vi "Patrick Excess-64.vi"() -> ()   [LabVIEW 2019]
panel:
  out "Boolean array 2":bool[][](array[boolean])=[[FALSE, TRUE, FALSE, FALSE, FALSE, FALSE, FALSE, TRUE, FALSE, FALSE, FALSE, TRUE, FALSE, FALSE, FALSE, FALSE, FALSE, FALSE, FALSE, FALSE, FALSE, FALSE, FALSE, FALSE, FALSE, FALSE, FALSE, FALSE, FALSE, FALSE, FALSE, FALSE], [FALSE, TRUE, FALSE, FALSE, FALSE, FALSE, FALSE, TRUE, FALSE, FALSE, TRUE, FALSE, FALSE, FALSE, FALSE, FALSE, FALSE, FALSE, FALSE, FALSE, FALSE, FALSE, FALSE, FALSE, FALSE, FALSE, FALSE, FALSE, FALSE, FALSE, FALSE, FALSE], [FALSE, TRUE, FALSE, FALSE, FALSE, FALSE, FALSE, TRUE, FALSE, FALSE, TRUE, TRUE, FALSE, FALSE, FALSE, FALSE, FALSE, FALSE, FALSE, FALSE, FALSE, FALSE, FALSE, FALSE, FALSE, FALSE, FALSE, FALSE, FALSE, FALSE, FALSE, FALSE], [TRUE, TRUE, FALSE, FALSE, FALSE, FALSE, FALSE, TRUE, FALSE, FALSE, FALSE, TRUE, FALSE, FALSE, FALSE, FALSE, FALSE, FALSE, FALSE, FALSE, FALSE, FALSE, FALSE, FALSE, FALSE, FALSE, FALSE, FALSE, FALSE, FALSE, FALSE, FALSE], [TRUE, TRUE, FALSE, FALSE, FALSE, FALSE, FALSE, TRUE, FALSE, FALSE, TRUE, FALSE, FALSE, FALSE, FALSE, FALSE, FALSE, FALSE, FALSE, FALSE, FALSE, FALSE, FALSE, FALSE, FALSE, FALSE, FALSE, FALSE, FALSE, FALSE, FALSE, FALSE], [TRUE, TRUE, FALSE, FALSE, FALSE, FALSE, FALSE, TRUE, FALSE, FALSE, TRUE, TRUE, FALSE, FALSE, FALSE, FALSE, FALSE, FALSE, FALSE, FALSE, FALSE, FALSE, FALSE, FALSE, FALSE, FALSE, FALSE, FALSE, FALSE, FALSE, FALSE, FALSE], [FALSE, TRUE, TRUE, FALSE, FALSE, FALSE, FALSE, FALSE, FALSE, TRUE, FALSE, FALSE, FALSE, FALSE, FALSE, FALSE, FALSE, FALSE, FALSE, FALSE, FALSE, FALSE, FALSE, FALSE, FALSE, FALSE, FALSE, FALSE, FALSE, FALSE, FALSE, TRUE], [FALSE, FALSE, TRUE, FALSE, FALSE, FALSE, FALSE, FALSE, FALSE, TRUE, FALSE, FALSE, TRUE, TRUE, FALSE, FALSE, TRUE, TRUE, FALSE, FALSE, TRUE, TRUE, FALSE, FALSE, TRUE, TRUE, FALSE, FALSE, TRUE, TRUE, FALSE, FALSE], [FALSE, FALSE, TRUE, FALSE, FALSE, FALSE, FALSE, FALSE, FALSE, TRUE, FALSE, TRUE, TRUE, FALSE, FALSE, TRUE, TRUE, FALSE, FALSE, TRUE, TRUE, FALSE, FALSE, TRUE, TRUE, FALSE, FALSE, TRUE, TRUE, FALSE, FALSE, TRUE], [FALSE, TRUE, FALSE, FALSE, FALSE, FALSE, FALSE, TRUE, FALSE, FALSE, FALSE, TRUE, TRUE, FALSE, TRUE, TRUE, FALSE, FALSE, TRUE, TRUE, FALSE, FALSE, TRUE, TRUE, FALSE, FALSE, TRUE, TRUE, FALSE, FALSE, TRUE, TRUE], [FALSE, FALSE, FALSE, FALSE, FALSE, FALSE, FALSE, FALSE, FALSE, FALSE, FALSE, FALSE, FALSE, FALSE, FALSE, FALSE, FALSE, FALSE, FALSE, FALSE, FALSE, FALSE, FALSE, FALSE, FALSE, FALSE, FALSE, FALSE, FALSE, FALSE, FALSE, FALSE], [FALSE, TRUE, FALSE, FALSE, FALSE, FALSE, FALSE, TRUE, FALSE, FALSE, FALSE, TRUE, FALSE, FALSE, FALSE, FALSE, FALSE, FALSE, FALSE, FALSE, FALSE, FALSE, FALSE, FALSE, FALSE, FALSE, FALSE, FALSE, FALSE, FALSE, FALSE, FALSE], [FALSE, TRUE, FALSE, FALSE, FALSE, FALSE, FALSE, TRUE, TRUE, FALSE, TRUE, FALSE, FALSE, FALSE, FALSE, FALSE, FALSE, FALSE, FALSE, FALSE, FALSE, FALSE, FALSE, FALSE, FALSE, FALSE, FALSE, FALSE, FALSE, FALSE, FALSE, FALSE], [FALSE, TRUE, FALSE, FALSE, FALSE, FALSE, TRUE, FALSE, FALSE, TRUE, TRUE, FALSE, FALSE, TRUE, FALSE, FALSE, FALSE, FALSE, FALSE, FALSE, FALSE, FALSE, FALSE, FALSE, FALSE, FALSE, FALSE, FALSE, FALSE, FALSE, FALSE, FALSE], [FALSE, TRUE, FALSE, FALSE, FALSE, FALSE, TRUE, TRUE, FALSE, FALSE, TRUE, TRUE, TRUE, TRUE, TRUE, FALSE, FALSE, FALSE, FALSE, FALSE, FALSE, FALSE, FALSE, TRUE, FALSE, FALSE, FALSE, FALSE, FALSE, FALSE, FALSE, FALSE], [FALSE, TRUE, FALSE, FALSE, FALSE, TRUE, FALSE, FALSE, FALSE, FALSE, TRUE, FALSE, FALSE, TRUE, TRUE, TRUE, FALSE, FALSE, FALSE, TRUE, FALSE, FALSE, FALSE, FALSE, FALSE, FALSE, FALSE, FALSE, FALSE, FALSE, FALSE, FALSE], [FALSE, TRUE, FALSE, FALSE, FALSE, TRUE, FALSE, TRUE, FALSE, FALSE, FALSE, TRUE, TRUE, FALSE, FALSE, FALSE, FALSE, TRUE, TRUE, FALSE, TRUE, FALSE, TRUE, FALSE, FALSE, FALSE, FALSE, FALSE, FALSE, FALSE, FALSE, FALSE]]
  out "?":u32=5642402 format="%064b"
  out "Boolean array":bool[](array[boolean])=[FALSE, TRUE, FALSE, FALSE, FALSE, TRUE, FALSE, TRUE, FALSE, FALSE, FALSE, TRUE, TRUE, FALSE, FALSE, FALSE, FALSE, TRUE, TRUE, FALSE, TRUE, FALSE, TRUE, FALSE, FALSE, FALSE, FALSE, FALSE, FALSE, FALSE, FALSE, FALSE]
  in  "Test numbers":u32[](array[numeric])=[1091567616, 1092616192, 1093664768, 3239051264, 3240099840, 3241148416, 1614807041, 541904076, 542742937, 1092301619, 0, 1091567616, 1101004800, 1113849856, 1128136960, 1143410688, 1159227904] format="%032b"
  out "Array":bool[][](array[boolean])=[[FALSE, FALSE, TRUE, TRUE, TRUE, TRUE, TRUE, FALSE], [FALSE, TRUE, FALSE, FALSE, FALSE, FALSE, FALSE, TRUE], [TRUE, FALSE, FALSE, FALSE, TRUE, FALSE, FALSE, TRUE], [FALSE, FALSE, TRUE, TRUE, FALSE, TRUE, TRUE, TRUE], [FALSE, TRUE, FALSE, FALSE, TRUE, FALSE, TRUE, TRUE], [TRUE, TRUE, FALSE, FALSE, FALSE, TRUE, TRUE, FALSE], [TRUE, FALSE, TRUE, FALSE, FALSE, TRUE, TRUE, TRUE], [TRUE, TRUE, TRUE, TRUE, FALSE, TRUE, FALSE, FALSE]]
  out "8 bytes":u8[](array[numeric])=[62, 65, 137, 55, 75, 198, 167, 244] format="%08b"
  out "result":dbl[](array[numeric])=[1.0, 2.0, 3.0, -1.0, -2.0, -3.0, 8.507061201264422e+37, inf, inf, 1.6999998092651367, nan, 1.0, 10.0, 100.0, 992.0625, 10000.0, 100000.0]
  # "https://boolean.klaasholwerda.nl/interface/bnf/gdsformat.html#datatypes"
  # "01000001000100000000000000000000 = 1\n01000001001000000000000000000000 = 2\n01000001001100000000000000000000 = 3\n11000001000100000000000000000000 = -1\n11000001001000000000000000000000 = -2\n11000001001100000000000000000000 = -3\n0100000010000000000000000000000 = 0 .5\n0100000010011001100110011001100 = 1 .6\n0100000010110011001100110011001 = 1 .7\n01000001000110000000000000000000 = 1.5\n01000001000110011001100110011001 = 1.6\n01000001000110110011001100110011 = 1.7\n00000000000000000000000000000000 = 0\n01000001000100000000000000000000 = 1\n01000001101000000000000000000000 = 10\n01000010011001000000000000000000 = 100\n01000011001111100000000100000000 = 1000\n01000100001001110001000000000000 = 10000\n01000101000110000110101000000000 = 100000"
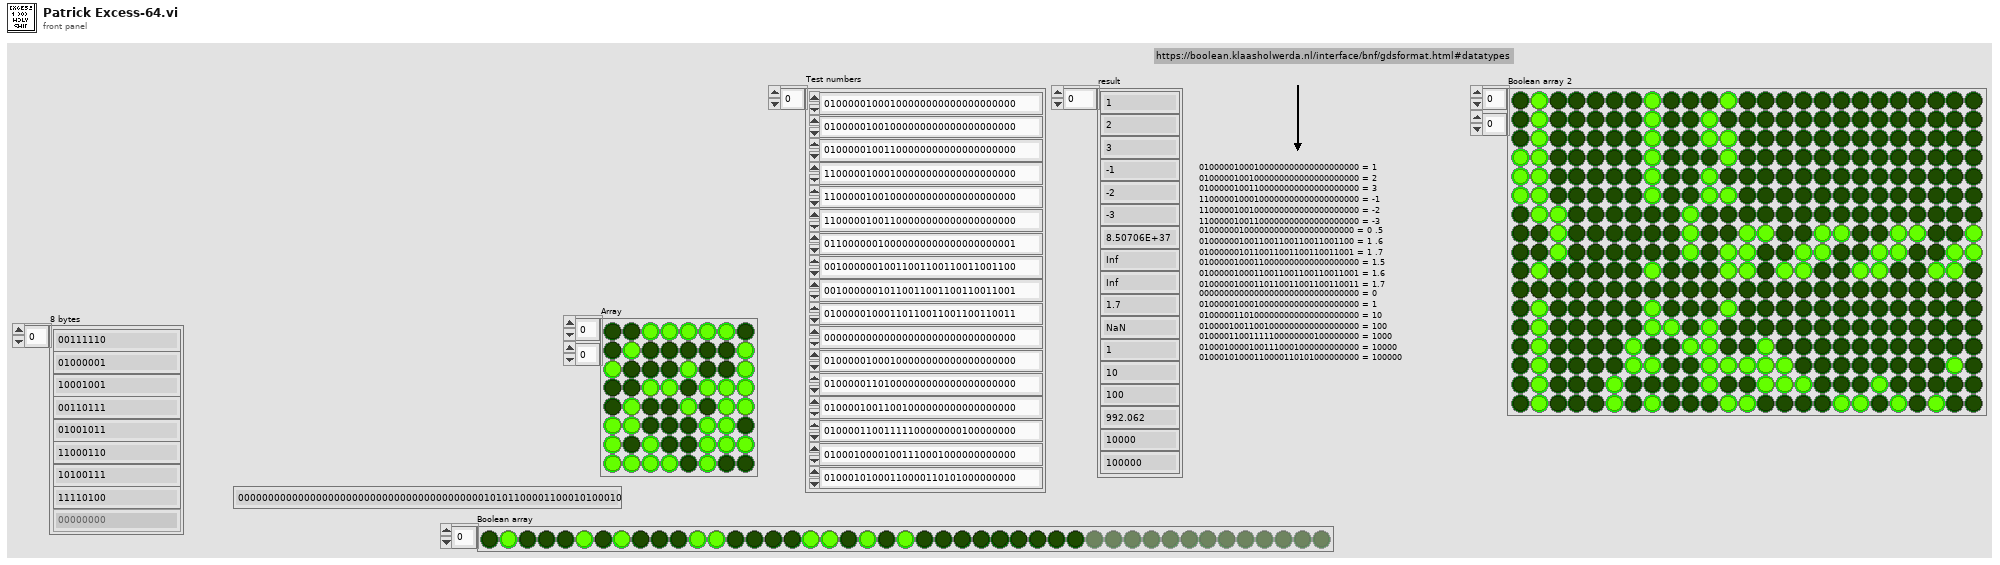
[diagram p1: front panel]
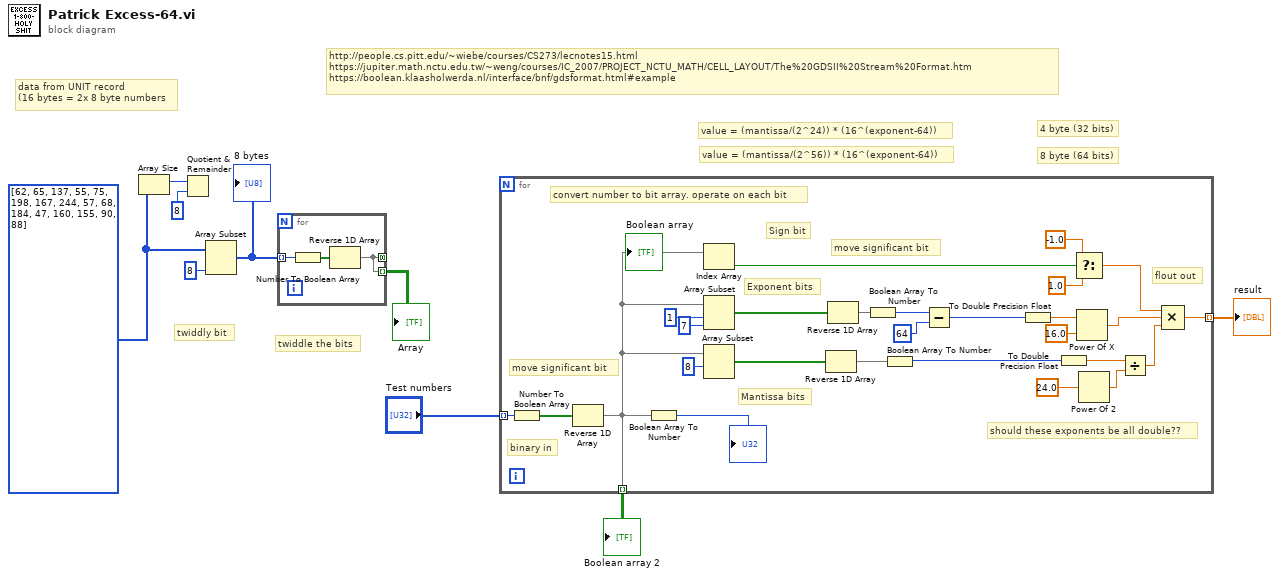
[diagram p0: block diagram]
diagram:
  w6 = u8[] [62, 65, 137, 55, 75, 198, 167, 244, 57, 68, 184, 47, 160, 155, 90, 88] ("Data")
  # "http://people.cs.pitt.edu/~wiebe/courses/CS273/lecnotes15.html\nhttps://jupiter.math.nctu.edu.tw/~weng/courses/IC_2007/PROJECT_NCTU_MATH/CELL_LAYOUT/The%20GDSII%20Stream%20Format.htm\nhttps://boolean.klaasholwerda.nl/interface/bnf/gdsformat.html#example"
  # "data from UNIT record\n(16 bytes = 2x 8 byte numbers"
  # "8 byte (64 bits)"
  # "4 byte (32 bits)"
  # "twiddly bit"
  # "twiddle the bits"
  # "value = (mantissa/(2^24)) * (16^(exponent-64))"
  # "value = (mantissa/(2^56)) * (16^(exponent-64))"
  n1 = Array Size(array=w6) -> (size(s)=w8:i32)
  n2 = Quotient & Remainder(x=w8, y=8 ("length")) -> ()  [unwired: 2 out]
  n3 = Array Subset(array=w6, length=8) -> (w4:u8[])  [unwired: 1 in]
  "8 bytes" <- w4
  n4 = for {
    tunnel: w4 -> [w12] mode=indexing
    tunnel: [w10] -> _ mode=concatenating
    tunnel: [w10] -> w3 mode=indexing
    n5 = Number To Boolean Array(number=w12) -> (Boolean array=w11:bool[])
    n6 = Reverse 1D Array(array=w11) -> (reversed array=w10:bool[])
  }
  "Array" <- w3
  n7 = for {
    tunnel: [w23] -> w7 mode=indexing
    tunnel: "Test numbers" -> [w19] mode=indexing
    tunnel: [w16] -> w1 mode=indexing
    # "flout out"
    # "binary in"
    # "should these exponents be all double??"
    # "move significant bit"
    # "Mantissa bits"
    # "move significant bit"
    # "convert number to bit array. operate on each bit"
    # "Exponent bits"
    # "Sign bit"
    n8 = Number To Boolean Array(number=w19) -> (Boolean array=w17:bool[])
    n9 = Reverse 1D Array(array=w17) -> (reversed array=w16:bool[])
    "Boolean array" <- w16
    n10 = Boolean Array To Number(Boolean array=w16) -> (number=→"?":u32)
    n11 = Index Array(array=w16) -> (element=w35:bool)  [unwired: 1 in]
    n12 = Array Subset(array=w16, index=1, length=7) -> (w15:bool[])
    n13 = Array Subset(array=w16, index=8) -> (w36:bool[])  [unwired: 1 in]
    n14 = Reverse 1D Array(array=w36) -> (reversed array=w22:bool[])
    n15 = Reverse 1D Array(array=w15) -> (reversed array=w21:bool[])
    n16 = Boolean Array To Number(Boolean array=w21) -> (number=w28:u32)
    n17 = Boolean Array To Number(Boolean array=w22) -> (number=w32:u32)
    n18 = Subtract(x=w28, y=u32 64) -> (x-y=w27:u32)
    n19 = To Double Precision Float(number=w27) -> (double precision float=w13:dbl)
    n20 = To Double Precision Float(number=w32) -> (double precision float=w14:dbl)
    n21 = Select(t=-1.0 ("x"), s=w35, f=1.0 ("x")) -> (s? t:f=w25:dbl)
    n22 = Power Of X(1:16.0 ("x"), 2:w13) -> (0:w18:dbl)
    n23 = Power Of 2(x=24.0) -> (2^x=w30:dbl)
    n24 = Divide(x=w14, y=w30) -> (x/y=w24:dbl)
    n25 = Compound Arithmetic op=MULTIPLY(w25, w18, w24) -> (w23:dbl)
  }
  "result" <- w7
  "Boolean array 2" <- w1
